vi "SavedSettingsWriteToINI.vi"(7 "Backup":bool=TRUE, 10 "Inifile path":path=path "C:/Users/osamu/Documents/LabVIEW Data/SettingsManager.ini", 11 "TreeControl in":refnum<vi>) -> ()   [LabVIEW 2019]
uses:
  <vilib>/Utility/config.llb/NI_LVConfig.lvlib
  <vilib>/Utility/config.llb/Write Key (I32).vi
  <vilib>/Utility/config.llb/Write Key (String).vi
  <vilib>/regexp/Match Regular Expression.xnode
  <vilib>/Utility/config.llb/Write Key (Boolean).vi
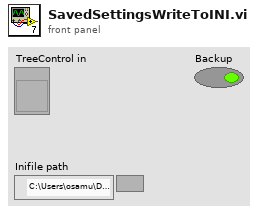
[diagram p1: front panel]
types:
  T1 = typedef "NI_LVConfig.lvlib/Config Data RefNum.ctl" = refnum<k1>
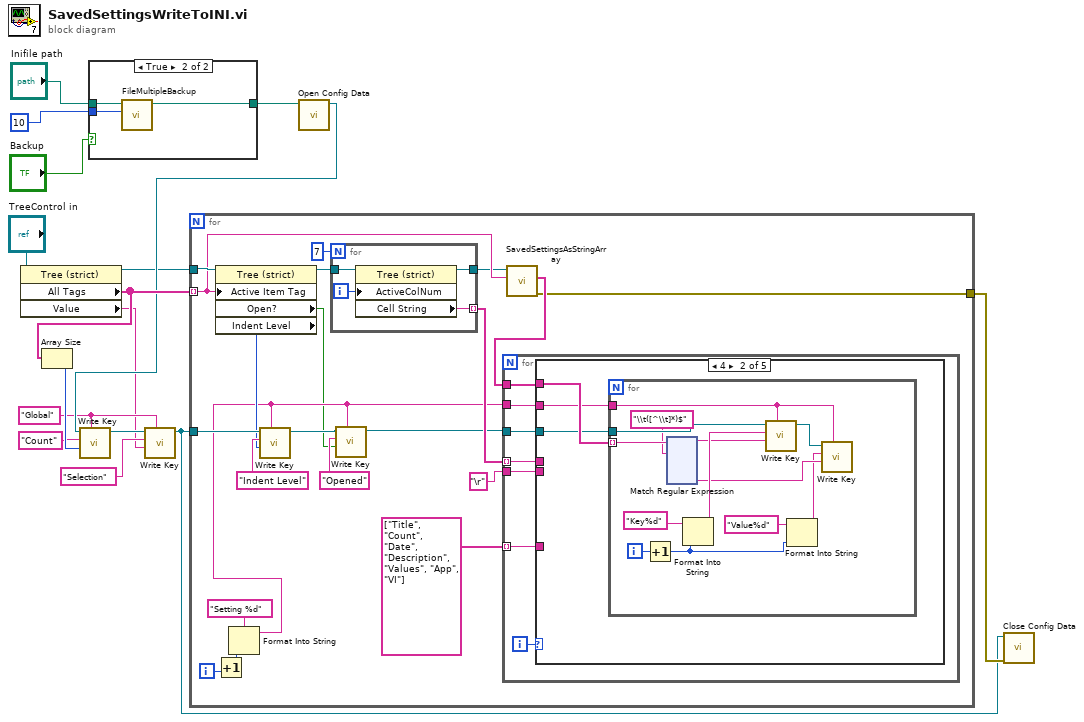
[diagram p0: block diagram]
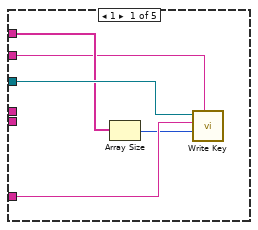
[diagram p3: hidden frame]
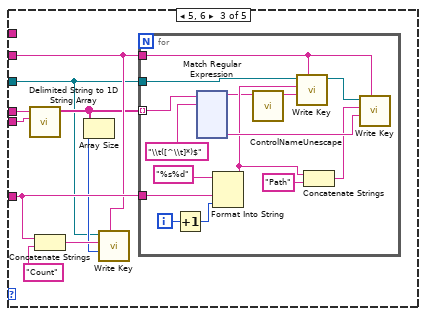
[diagram p4: hidden frame]
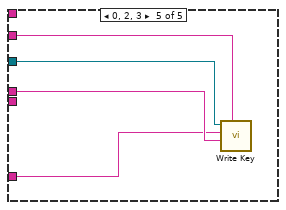
[diagram p6: hidden frame]
diagram:
  w4 = "Global" ("section")
  n1 = property class="Tree (strict)"(reference="TreeControl in") -> (reference out=w12:refnum<vi>, "All Tags"=w15:string[], "Value"=w2:string)  [unwired: 1 in, 1 out]
  n2 = Array Size(array=w15) -> (size(s)=w16:i32)
  n3 = case shown="True" "Backup" {
    tunnel: "Inifile path" -> [w17 w20]
    tunnel: [w17 w19] -> w8
    tunnel: 10 ("Number of Backup") -> [_ w18]
    frame False {
    }
    frame True {
      n4 = call "FileMultipleBackup.vi"("Number of Backups"=w18, "File path"=w20) -> ("File path out"=w19:path)  [unwired: 9 in]
    }
  }
  n5 = call <vilib>:"Open Config Data.vi"("configuration file path"=w8) -> ("refnum"=w13:T1)  [unwired: 8 in, 2 out]
  n6 = call-poly <vilib>:"Write Key.vi"("section"=w4, "value"=w16, "key"="Count", "refnum"=w13) -> ("refnum out"=w5:T1)  [unwired: 5 in, 2 out]
  n7 = call-poly <vilib>:"Write Key.vi"("section"=w4, "value"=w2, "key"="Selection", "refnum"=w5) -> ("refnum out"=w3:T1)  [unwired: 5 in, 2 out]
  n8 = for {
    tunnel: w15 -> [w32] mode=indexing
    tunnel: w12 -> [w41]
    tunnel: w3 -> [w38]
    tunnel: [w28] -> w10
    i -> [w37]
    n9 = property class="Tree (strict)"(reference=w41, "Active Item Tag"=w32) -> (reference out=w39:refnum<vi>, "Open?"=w21:bool, "Indent Level"=w26:i32)  [unwired: 1 in, 1 out]
    n10 = Increment(x=w37) -> (x+1=w35:i32)
    n11 = Format Into String(format string="Setting %d", w35) -> (resulting string=w22:string)  [unwired: 2 in, 1 out]
    n12 = call-poly <vilib>:"Write Key.vi"("section"=w22, "value"=w26, "key"="Indent Level", "refnum"=w38) -> ("refnum out"=w24:T1)  [unwired: 5 in, 2 out]
    n13 = for {
      N: 7 -> [_]
      tunnel: w39 -> [w339]
      tunnel: [w337] -> w33 mode=indexing
      tunnel: [w336] -> w31
      i -> [w338]
      n14 = property class="Tree (strict)"(reference=w339, "ActiveColNum"=w338) -> (reference out=w336:refnum<vi>, "Cell String"=w337:string)  [unwired: 1 in, 1 out]
    }
    n15 = call-poly <vilib>:"Write Key.vi"("section"=w22, "value"=w21, "key"="Opened", "refnum"=w24) -> ("refnum out"=w23:T1)  [unwired: 5 in, 2 out]
    n16 = call "SavedSettingsAsStringArray.vi"("Tag"=w32, "SavedSettings in"=w31) -> ("error out"=w28:errorcluster, "Selection"=w30:string[])  [unwired: 5 in, 3 out]
    n17 = for {
      tunnel: w33 -> [w46] mode=indexing
      tunnel: string[] ["Title", "Count", "Date", "Description", "Values", "App", "VI"] -> [w45] mode=indexing
      tunnel: w22 -> [w47]
      tunnel: w23 -> [w44]
      tunnel: w30 -> [w43]
      tunnel: "\r" ("delimiter") -> [w42]
      i -> [w48]
      n18 = case shown="4" w48 {
        tunnel: w47 -> [w49 w55 w194 _ w335]
        tunnel: w46 -> [_ _ w197 _ w334]
        tunnel: w45 -> [w52 _ w196 _ w333]
        tunnel: w44 -> [w53 w54 w191 _ w332]
        tunnel: w43 -> [w50 w56 _ _ _]
        tunnel: w42 -> [_ _ w190 _ _]
        frame 1 {
          n19 = Array Size(array=w50) -> (size(s)=w51:i32)
          n20 = call-poly <vilib>:"Write Key.vi"("section"=w49, "value"=w51, "key"=w52, "refnum"=w53) -> ()  [unwired: 5 in, 3 out]
        }
        frame 4 {
          n21 = for {
            tunnel: w56 -> [w67] mode=indexing
            tunnel: w55 -> [w58]
            tunnel: w54 -> [w66]
            i -> [w69]
            n22 = Increment(x=w69) -> (x+1=w62:i32)
            n23 = xnode "Match Regular Expression"("input string"=w67, "regular expression"="\\t([^\\t]*)$" ("input string")) -> ("before match"=w57:string, "submatch 1"=w64:string)  [unwired: 4 in, 4 out]
            n24 = Format Into String(format string="Key%d", w62) -> (resulting string=w65:string)  [unwired: 2 in, 1 out]
            n25 = call-poly <vilib>:"Write Key.vi"("section"=w58, "value"=w57, "key"=w65, "refnum"=w66) -> ("refnum out"=w60:T1)  [unwired: 5 in, 2 out]
            n26 = Format Into String(format string="Value%d", w62) -> (resulting string=w61:string)  [unwired: 2 in, 1 out]
            n27 = call-poly <vilib>:"Write Key.vi"("section"=w58, "value"=w64, "key"=w61, "refnum"=w60) -> ()  [unwired: 5 in, 3 out]
          }
        }
        frame 5, 6 {
          n28 = call <vilib>:"Delimited String to 1D String Array.vi"("delimiter"=w190, "delimited string"=w197) -> ("string array"=w193:string[])  [unwired: 9 in]
          n29 = Concatenate Strings(w196, "Count" ("string")) -> (w195:string)
          n30 = Array Size(array=w193) -> (size(s)=w192:i32)
          n31 = call-poly <vilib>:"Write Key.vi"("section"=w194, "value"=w192, "key"=w195, "refnum"=w191) -> ()  [unwired: 5 in, 3 out]
          n32 = for {
            tunnel: w193 -> [w210] mode=indexing
            tunnel: w194 -> [w205]
            tunnel: w191 -> [w209]
            tunnel: w196 -> [w204]
            i -> [w212]
            n33 = Increment(x=w212) -> (x+1=w203:i32)
            n34 = xnode "Match Regular Expression"("input string"=w210, "regular expression"="\\t([^\\t]*)$" ("input string")) -> ("before match"=w199:string, "submatch 1"=w208:string)  [unwired: 4 in, 4 out]
            n35 = Format Into String(format string="%s%d", w204, w203) -> (resulting string=w201:string)  [unwired: 2 in, 1 out]
            n36 = call "ControlNameUnescape.vi"("escaped string"=w199) -> ("label"=w198:string)  [unwired: 10 in]
            n37 = call-poly <vilib>:"Write Key.vi"("section"=w205, "value"=w198, "key"=w201, "refnum"=w209) -> ("refnum out"=w207:T1)  [unwired: 5 in, 2 out]
            n38 = Concatenate Strings(w201, "Path" ("string")) -> (w202:string)
            n39 = call-poly <vilib>:"Write Key.vi"("section"=w205, "value"=w208, "key"=w202, "refnum"=w207) -> ()  [unwired: 5 in, 3 out]
          }
        }
        frame Default {
        }
        frame 0, 2, 3 {
          n40 = call-poly <vilib>:"Write Key.vi"("section"=w335, "value"=w334, "key"=w333, "refnum"=w332) -> ()  [unwired: 5 in, 3 out]
        }
      }
    }
  }
  n41 = call <vilib>:"Close Config Data.vi"("error in (no error)"=w10, "refnum"=w3) -> ()  [unwired: 8 in, 2 out]
